vi "Source Close.vi"(8 "error in":errorcluster, 11 "src in":T1={"type"=enum."Tektronix AFG3101C", "afg"={"VISA"="", "const"=0.0, "gen DC"=FALSE, "ext ref"=FALSE}, "cDAQ dds"={"device"="", "channels"=[], "mclk source"="", "mclk [Hz]"=0.0, "fs [Hz]"=0.0, "block [s]"=0.0, "buf [s]"=0.0, "task"="", "cmd queue"=refnum, "proc ref"=refnum, "smpl clock out"="/cDAQ3/PFI0", "export smpl clock"=FALSE, "DC ofs [V]"=[], "timebase source"="", "timebase mode"=enum."Local"}, "gain [V/A]"=1.0, "F5xxx session"={"VISA"="", "mode"=enum."AC voltage", "Earth on"=FALSE, "Ext ref lock"=FALSE}} {"cDAQ dds"."channels" min=0 step=1}) -> (0 "error out":errorcluster, 3 "src out":T1={"type"=enum."Tektronix AFG3101C", "afg"={"VISA"="", "const"=0.0, "gen DC"=FALSE, "ext ref"=FALSE}, "cDAQ dds"={"device"="", "channels"=[], "mclk source"="", "mclk [Hz]"=0.0, "fs [Hz]"=0.0, "block [s]"=0.0, "buf [s]"=0.0, "task"="", "cmd queue"=refnum, "proc ref"=refnum, "smpl clock out"="/cDAQ3/PFI0", "export smpl clock"=FALSE, "DC ofs [V]"=[], "timebase source"="", "timebase mode"=enum."Local"}, "gain [V/A]"=1.0, "F5xxx session"={"VISA"="", "mode"=enum."AC voltage", "Earth on"=FALSE, "Ext ref lock"=FALSE}} {"cDAQ dds"."channels" min=0 step=1})   [LabVIEW 2020]
doc: "Close source."
uses:
  Source Session.ctl
  Source Type.ctl
  drivers/AFG3101C/AFG3101C Session.ctl
  drivers/cDAQ DDS/cDAQ DDS Session.ctl
  drivers/cDAQ DDS/cDAQ DDS Setup.ctl
  drivers/cDAQ DDS/cDAQ DDS Timebase Mode.ctl
  drivers/Fluke 5XXX/top_lev/F5xxx_session.ctl
  drivers/Fluke 5XXX/top_lev/F5xxx_output_mode.ctl
  <vilib>/Instr/_visa.llb/VISA GPIB Control REN Mode.ctl
  drivers/AFG3101C/Tektronix AFG 3000 Series.lvlib
  <vilib>/Utility/error.llb/Error Cluster From Error Code.vi
  <vilib>/ErrorRing/Error Ring.xnode
  drivers/Agilent 33XXX Series/Agilent 33XXX Series.lvlib
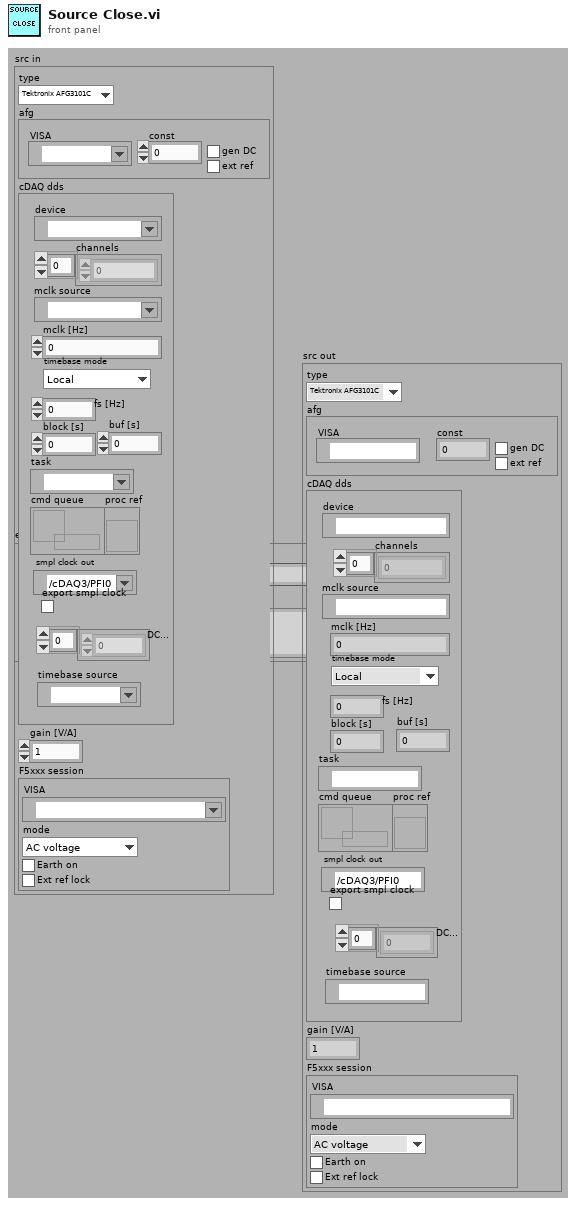
[diagram p1: front panel]
types:
  T1 = typedef "Source Session.ctl" = cluster{"type":T2, "afg":T3, "cDAQ dds":T4, "gain [V/A]":dbl, "F5xxx session":T6}
  T2 = typedef "Source Type.ctl" = enum16{"Tektronix AFG3101C", "cDAQ DAC", "Fluke 5xxx", "Agilent 33120A", "dummy"}
  T3 = typedef "AFG3101C Session.ctl" = cluster{"VISA":refnum<visa-resource-name>, "const":dbl, "gen DC":bool, "ext ref":bool}
  T4 = typedef "cDAQ DDS Session.ctl" = cluster{"device":tag, "channels":i32[], "mclk source":tag, "mclk [Hz]":dbl, "fs [Hz]":dbl, "block [s]":dbl, "buf [s]":dbl, "task":refnum<k21>, "cmd queue":refnum<queue>, "proc ref":refnum<vi>, "smpl clock out":tag, "export smpl clock":bool, "DC ofs [V]":dbl[], "timebase source":tag, "timebase mode":T5}
  T5 = typedef "cDAQ DDS Timebase Mode.ctl" = enum16{"Local", "Take from ADC (e.g. NI 9238)", "Other source"}
  T6 = typedef "F5xxx_session.ctl" = cluster{"VISA":refnum<visa-resource-name>, "mode":T7, "Earth on":bool, "Ext ref lock":bool}
  T7 = typedef "F5xxx_output_mode.ctl" = enum16{"AC voltage", "AC current"}
  T8 = typedef "VISA GPIB Control REN Mode.ctl" = u16
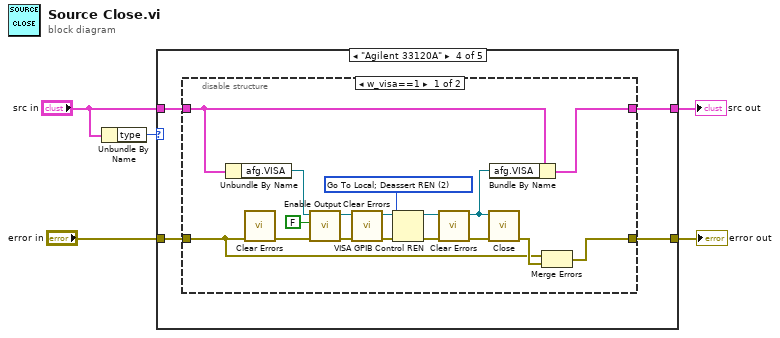
[diagram p0: block diagram]
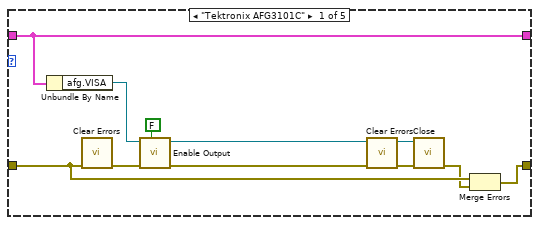
[diagram p2: hidden frame]
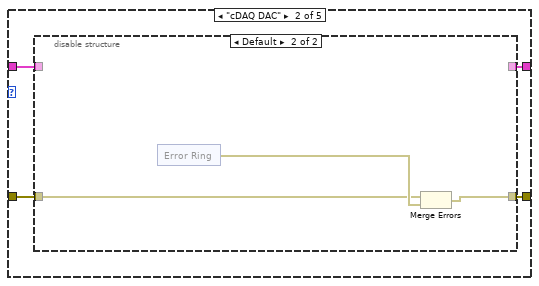
[diagram p3: hidden frame]
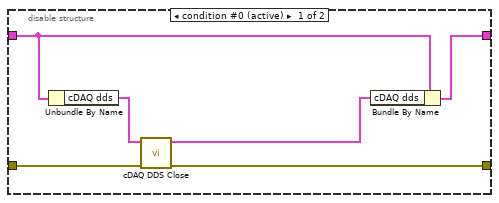
[diagram p4: hidden frame]
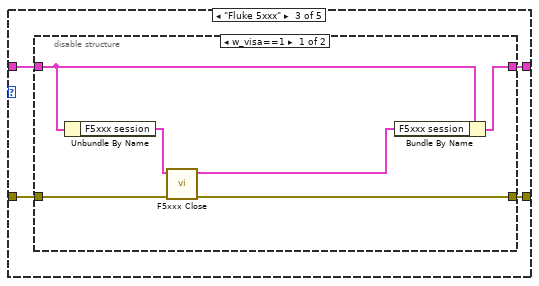
[diagram p5: hidden frame]
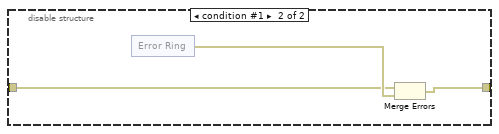
[diagram p6: hidden frame]
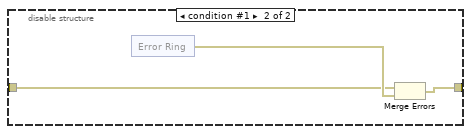
[diagram p7: hidden frame]
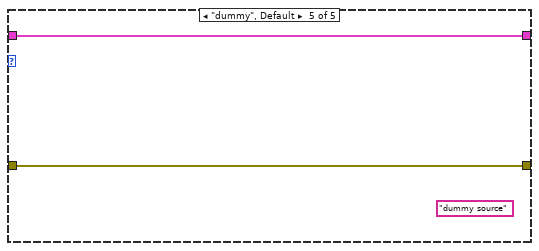
[diagram p8: hidden frame]
diagram:
  n1 = Unbundle By Name("src in") -> ("type"=w4:T2)
  n2 = case shown="\"Agilent 33120A\"" w4 {
    tunnel: "src in" -> [w6 w18 w36 w54 w80]
    tunnel: "error in" -> [w10 w19 w37 w55 w79]
    tunnel: [w8 w17 w35 w53 w79] -> w2
    tunnel: [w6 w16 w34 w52 w80] -> w1
    frame "Tektronix AFG3101C" {
      n3 = Unbundle By Name(w6) -> ("afg.VISA"=w15:refnum<visa-resource-name>)
      n4 = call <vilib>:"Clear Errors.vi"("error in (no error)"=w10) -> ("error out"=w11:errorcluster)  [unwired: 5 in, 1 out]
      n5 = call "Enable Output.vi"("Enable Output (T: Enable)"=FALSE, "error in (no error)"=w11, "VISA resource name"=w15) -> ("error out"=w13:errorcluster, "VISA resource name out"=w14:refnum<visa-resource-name>)  [unwired: 7 in]
      n6 = call <vilib>:"Clear Errors.vi"("error in (no error)"=w13) -> ("error out"=w12:errorcluster)  [unwired: 5 in, 1 out]
      n7 = call "Close.vi"("error in (no error)"=w12, "VISA resource name"=w14) -> ("error out"=w9:errorcluster)  [unwired: 9 in]
      n8 = Merge Errors(w10, w9) -> (w8:errorcluster)
    }
    frame "cDAQ DAC" {
      n9 = disable-structure shown="Default" {
        disable-tunnel: w19 -> [w25 w26]
        disable-tunnel: w18 -> [w23 _]
        disable-tunnel: [w21 w27] -> w17
        disable-tunnel: [w20 _] -> w16
        frame condition #0 (active) {
          n10 = Unbundle By Name(w23) -> ("cDAQ dds"=w24:T4)
          n11 = call "cDAQ DDS Close.vi"("error in"=w25, "cdaq session in"=w24) -> ("error out"=w21:errorcluster, "cdaq session out"=w22:T4)  [unwired: 8 in]
          n12 = Bundle By Name(cluster=w23, "cDAQ dds"=w22) -> (w20:T1)
        }
        frame condition #1 {
          n13 = xnode "Error Ring"() -> ("error out"=w28:errorcluster)
          n14 = Merge Errors(w26, w28) -> (w27:errorcluster)
        }
      }
    }
    frame "Fluke 5xxx" {
      n15 = disable-structure shown="w_visa==1" {
        disable-tunnel: w37 -> [w43 w44]
        disable-tunnel: w36 -> [w42 _]
        disable-tunnel: [w40 w45] -> w35
        disable-tunnel: [w39 _] -> w34
        frame condition #0 (active) {
          n16 = Unbundle By Name(w42) -> ("F5xxx session"=w38:T6)
          n17 = call "F5xxx Close.vi"("error in (no error)"=w43, "session in"=w38) -> ("error out"=w40:errorcluster, "session out"=w41:T6)  [unwired: 8 in]
          n18 = Bundle By Name(cluster=w42, "F5xxx session"=w41) -> (w39:T1)
        }
        frame condition #1 {
          n19 = xnode "Error Ring"() -> ("error out"=w46:errorcluster)
          n20 = Merge Errors(w44, w46) -> (w45:errorcluster)
        }
      }
    }
    frame "Agilent 33120A" {
      n21 = disable-structure shown="w_visa==1" {
        disable-tunnel: w55 -> [w63 w71]
        disable-tunnel: w54 -> [w70 _]
        disable-tunnel: [w56 w72] -> w53
        disable-tunnel: [w69 _] -> w52
        frame condition #0 (active) {
          w60 = T8 2 items=["Deassert REN", "Assert REN", "Go To Local; Deassert REN ", "Assert REN; Address Device", "Local Lockout (Addressed Devices)", "Local Lockout (This Device)", "Go To Local"] ("Mode")
          n22 = Unbundle By Name(w70) -> ("afg.VISA"=w68:refnum<visa-resource-name>)
          n23 = call <vilib>:"Clear Errors.vi"("error in (no error)"=w63) -> ("error out"=w67:errorcluster)  [unwired: 5 in, 1 out]
          n24 = call "Enable Output.vi"("error in (no error)"=w67, "Enable Output  (T: Enable)"=FALSE, "VISA resource name"=w68) -> ("error out"=w65:errorcluster, "VISA resource name out"=w61:refnum<visa-resource-name>)  [unwired: 7 in]
          n25 = call <vilib>:"Clear Errors.vi"("error in (no error)"=w65) -> ("error out"=w62:errorcluster)  [unwired: 5 in, 1 out]
          n26 = VISA GPIB Control REN(8:w62, 10:w60, 11:w61) -> (0:w59:errorcluster, 3:w57:refnum<visa-resource-name>)
          n27 = call <vilib>:"Clear Errors.vi"("error in (no error)"=w59) -> ("error out"=w58:errorcluster)  [unwired: 5 in, 1 out]
          n28 = call "Close.vi"("error in (no error)"=w58, "VISA resource name"=w57) -> ("error out"=w64:errorcluster)  [unwired: 9 in]
          n29 = Bundle By Name(cluster=w70, "afg.VISA"=w57) -> (w69:T1)
          n30 = Merge Errors(w63, w64) -> (w56:errorcluster)
        }
        frame condition #1 {
          n31 = xnode "Error Ring"() -> ("error out"=w73:errorcluster)
          n32 = Merge Errors(w71, w73) -> (w72:errorcluster)
        }
      }
    }
    frame "dummy", Default {
      (unwired) "dummy source" ("idn string")
    }
  }
  "error out" <- w2
  "src out" <- w1
